vi "Create All Message Queues.vi"(8 "error in (no error)":errorcluster, 11 "Message Queues":T1) -> (0 "error out":errorcluster, 3 "Message Queues out":T1)   [LabVIEW 2017, in "WaveformGenerator.lvlib" / "MessageQueue.lvlib"]
doc: "This VI creates and initializes all the message queues for your application. If your application requires more than one message queue, right-click the \"Message Queues\" constant above and select Open Type Def. Add the new Message Queue(s) to the type definition, then initialize them in this VI."
uses:
  MessageQueue.lvlib
  All Message Queues.ctl
  Message Cluster.ctl
  Enqueue Message (Single).vi
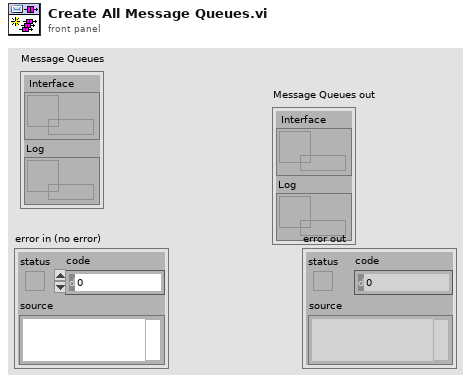
[diagram p1: front panel]
types:
  T1 = typedef "WaveformGenerator.lvlib/MessageQueue.lvlib/All Message Queues.ctl" = cluster{" Interface":refnum<queue>, "Log":refnum<queue>}
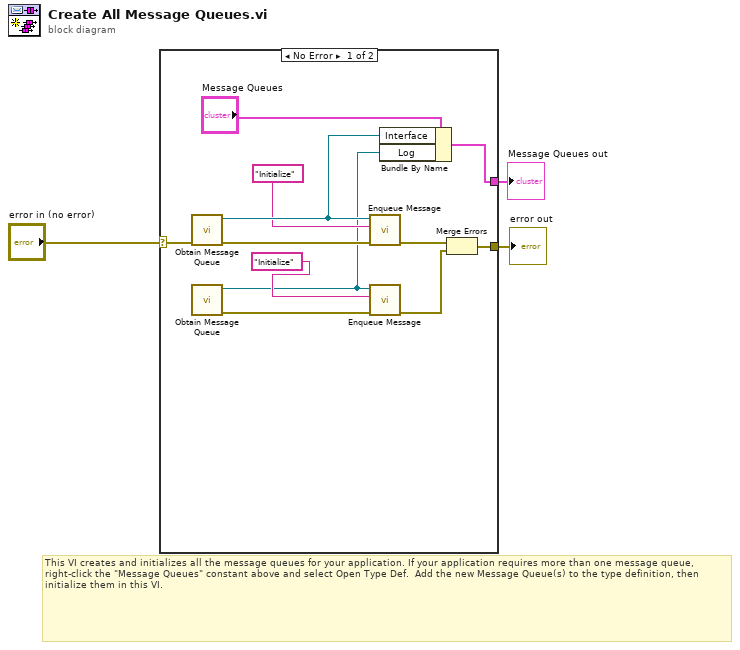
[diagram p0: block diagram]
diagram:
  # "This VI creates and initializes all the message queues for your application. If your application requires more than one message queue, right-click the \"Message Queues\" constant above and select Open Type Def.  Add the new Message Queue(s) to the type definition, then initialize them in this VI."
  n1 = case shown="No Error" "error in (no error)" {
    selector: "error in (no error)" -> [w9 w16]
    tunnel: [w11 w16] -> w3
    tunnel: [w14 _] -> w2
    frame No Error {
      n2 = call "Obtain Message Queue.vi"("error in (no error)"=w9) -> ("error out"=w13:errorcluster, "Message Queue"=w10:refnum<queue>)  [unwired: 9 in]
      n3 = call "Obtain Message Queue.vi"() -> ("error out"=w7:errorcluster, "Message Queue"=w4:refnum<queue>)  [unwired: 10 in]
      n4 = call-poly "Enqueue Message.vi"("error in (no error)"=w13, "Message"="Initialize", "Message Queue"=w10) -> ("error out"=w12:errorcluster)  [unwired: 7 in, 1 out]
      n5 = call-poly "Enqueue Message.vi"("error in (no error)"=w7, "Message"="Initialize", "Message Queue"=w4) -> ("error out"=w5:errorcluster)  [unwired: 7 in, 1 out]
      n6 = Bundle By Name(cluster="Message Queues", "Interface"=w10, "Log"=w4) -> (w14:T1)
      n7 = Merge Errors(w12, w5) -> (w11:errorcluster)
    }
    frame Error {
    }
  }
  "Message Queues out" <- w2
  "error out" <- w3
